vi "dbc-FIND-ALL-FRAME-SIGNALS.vi"(8 "error in (no error)":errorcluster, 10 "tag":string, 11 "dbc in":refnum<class "dbc.lvclass">) -> (0 "error out":errorcluster, 2 "tag.Array":string[](array[string]), 3 "dbc out":refnum<class "dbc.lvclass">)   [LabVIEW 2015, in "dbc.lvclass"]
uses:
  dbc.lvclass
  dbc.lvclass/dbc.ctl
  read-tree-ref.vi
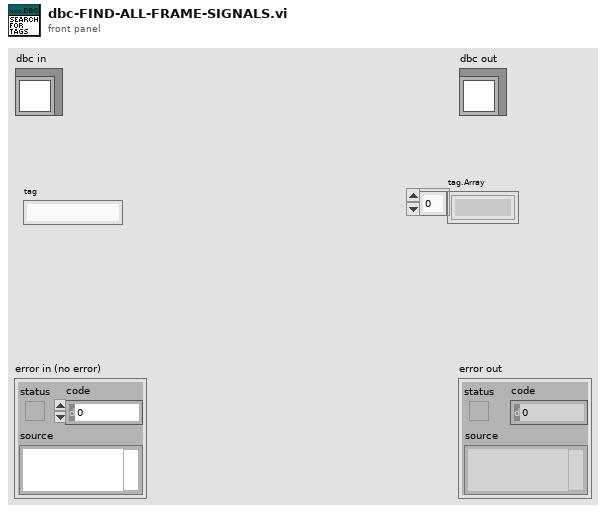
[diagram p1: front panel]
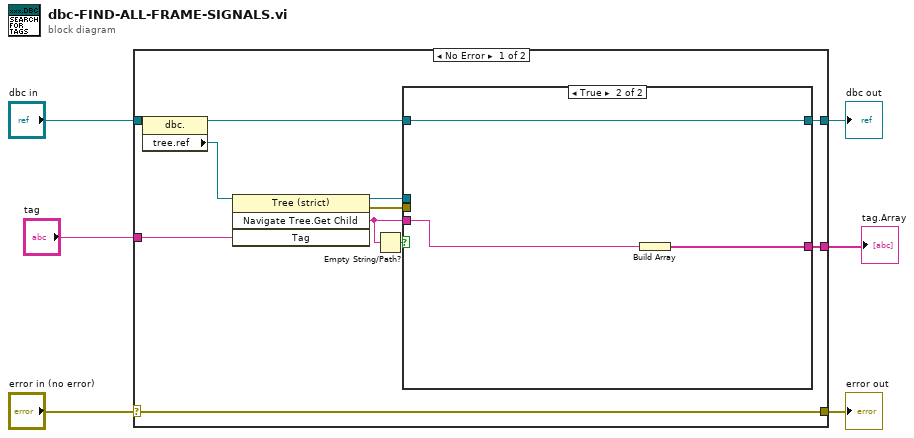
[diagram p0: block diagram]
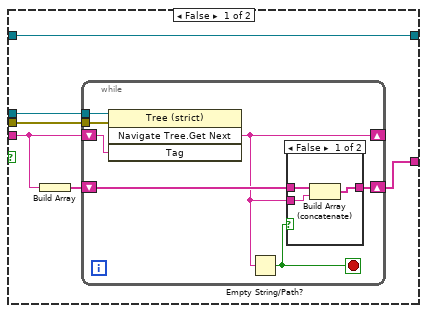
[diagram p2: hidden frame]
diagram:
  n1 = case shown="No Error" "error in (no error)" {
    selector: "error in (no error)" -> [w16 w39]
    tunnel: [w16 w39] -> w5
    tunnel: [w8 w38] -> w3
    tunnel: "dbc in" -> [w17 w38]
    tunnel: "tag" -> [w7 _]
    tunnel: [w15 _] -> w1
    frame No Error {
      n2 = property class="dbc."(reference=w17) -> (reference out=w9:refnum<class "dbc.lvclass">, "tree.ref"=w14:refnum<vi>)  [unwired: 1 in, 1 out]
      n3 = invoke class="Tree (strict)" method="Navigate Tree.Get Child"(reference=w14, "Tag"=w7) -> (reference out=w13:refnum<vi>, error out=w12:errorcluster, "Navigate Tree:Get Child"=w10:string)  [unwired: 2 in, 1 out]
      n4 = Empty String/Path?(string/path=w10) -> (empty?=w11:bool)
      n5 = case shown="True" w11 {
        tunnel: w13 -> [w23 _]
        tunnel: w12 -> [w22 _]
        tunnel: w10 -> [w19 w37]
        tunnel: [w18 w36] -> w15
        tunnel: w9 -> [w21 w35]
        tunnel: [w21 w35] -> w8
        frame False {
          n6 = Build Array(w19) -> (w20:string[])
          n7 = while {
            tunnel: w23 -> [w30]
            tunnel: w22 -> [w29]
            shift-right: [w24] -> _
            shift-left: w19 -> [w28]
            shift-right: [w26] -> w18
            shift-left: w20 -> [w27]
            stop <- w25 stop-if-true
            n8 = invoke class="Tree (strict)" method="Navigate Tree.Get Next"(reference=w30, error in=w29, "Tag"=w28) -> ("Navigate Tree:Get Next Item"=w24:string)  [unwired: 1 in, 3 out]
            n9 = Empty String/Path?(string/path=w24) -> (empty?=w25:bool)
            n10 = case shown="False" w25 {
              tunnel: w27 -> [w33 w34]
              tunnel: [w32 w34] -> w26
              tunnel: w24 -> [w31 _]
              frame False {
                n11 = Build Array (concatenate)(w33, w31) -> (w32:string[])
              }
              frame True {
              }
            }
          }
        }
        frame True {
          n12 = Build Array(w37) -> (w36:string[])
        }
      }
    }
    frame Error {
    }
  }
  "error out" <- w5
  "dbc out" <- w3
  "tag.Array" <- w1
